vi "uploadBLE.vi"(11 "Queue in":refnum<queue>) -> ()   [LabVIEW 2022 SP3]
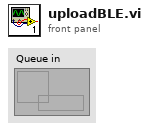
[diagram p1: front panel]
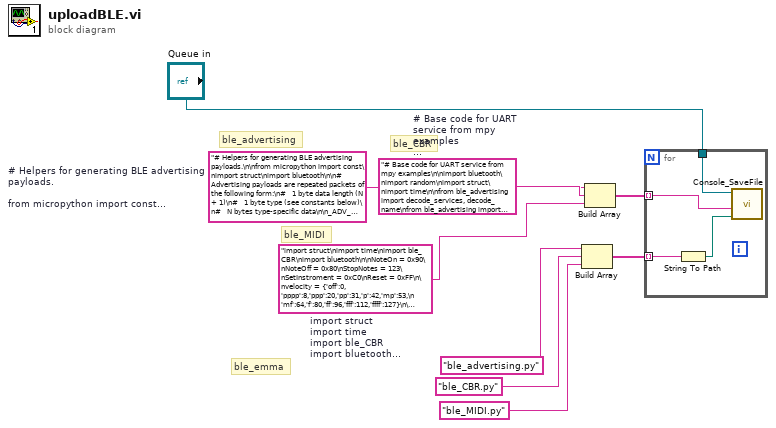
[diagram p0: block diagram]
diagram:
  w8 = "import struct\nimport time\nimport ble_CBR\nimport bluetooth\n\nNoteOn = 0x90\nNoteOff = 0x80\nStopNotes = 123\nSetInstroment = 0xC0\nReset = 0xFF\n\nvelocity = {'off':0, 'pppp':8,'ppp':20,'pp':31,'p':42,'mp':53,\n    'mf':64,'f':80,'ff':96,'fff':112,'ffff':127}\n\ninstruments = {'Acoustic Grand Piano':0,'Bright Acoustic Piano':1,'Electric Grand Piano':2,'Honky-tonk Piano':3,'Rhodes Piano':4,'Chorused Piano':5,'Harpsichord':6,'Clavinet':7,'Celesta':8,'Glockenspiel':9,'Music box':10,'Vibraphone':11,'Marimba':12,'Xylophone':13,'Tubular Bells':14,'Dulcimer':15,'Hammond Organ':16,'Percussive Organ':17,'Rock Organ':18,'Church Organ':19,\n    'Reed Organ':20,'Accordion':21,'Harmonica':22,'Tango Accordion':23,'Acoustic Guitar (nylon)':24,'Acoustic Guitar (steel)':25,'Electric Guitar (jazz)':26,'Electric Guitar (clean)':27,'Electric Guitar (muted)':28,'Overdriven Guitar':29,'Distortion Guitar':30,'Guitar Harmonics':31,'Acoustic Bass':32,'Electric Bass (finger)':33,'Electric Bass (pick)':34,'Fretless Bass':35,\n    'Slap Bass 1':36,'Slap Bass 2':37,'Synth Bass 1':38,'Synth Bass 2':39,'Violin':40,'Viola':41,'Cello':42,'Contrabass':43,'Tremolo Strings':44,'Pizzicato Strings':45,'Orchestral Harp':46,'Timpani':47,'String Ensemble 1':48,'String Ensemble 2':49,'Synth Strings 1':50,'Synth Strings 2':51,'Choir Aahs':52,'Voice Oohs':53,'Synth Voice':54,'Orchestra Hit':55,'Trumpet':56,\n    'Trombone':57,'Tuba':58,'Muted Trumpet':59,'French Horn':60,'Brass Section':61,'Synth Brass 1':62,'Synth Brass 2':63,'Soprano Sax':64,'Alto Sax':65,'Tenor Sax':66,'Baritone Sax':67,'Oboe':68,'English Horn':69,'Bassoon':70,'Clarinet':71,'Piccolo':72,'Flute':73,'Recorder':74,'Pan Flute':75,'Bottle Blow':76,'Shakuhachi':77,'Whistle':78,'Ocarina':79,'Lead 1 (square)':80,\n    'Lead 2 (sawtooth)':81,'Lead 3 (calliope lead)':82,'Lead 4 (chiffer lead)':83,'Lead 5 (charang)':84,'Lead 6 (voice)':85,'Lead 7 (fifths)':86,'Lead 8 (brass + lead)':87,'Pad 1 (new age)':88,'Pad 2 (warm)':89,'Pad 3 (polysynth)':90,'Pad 4 (choir)':91,'Pad 5 (bowed)':92,'Pad 6 (metallic)':93,'Pad 7 (halo)':94,'Pad 8 (sweep)':95,'FX 1 (rain)':96,'FX 2 (soundtrack)':97,\n    'FX 3 (crystal)':98,'FX 4 (atmosphere)':99,'FX 5 (brightness)':100,'FX 6 (goblins)':101,'FX 7 (echoes)':102,'FX 8 (sci-fi)':103,'Sitar':104,'Banjo':105,'Shamisen':106,'Koto':107,'Kalimba':108,'Bagpipe':109,'Fiddle':110,'Shana':111,'Tinkle Bell':112,'Agogo':113,'Steel Drums':114,'Woodblock':115,'Taiko Drum':116,'Melodic Tom':117,'Synth Drum':118,'Reverse Cymbal':119,\n    'Guitar Fret Noise':120,'Breath Noise':121,'Seashore':122,'Bird Tweet':123,'Telephone Ring':124,'Helicopter':125,'Applause':126,'Gunshot':127}\n\nclass MIDI_Player:\n    def __init__(self, name = 'MySpike'):\n        ble = bluetooth.BLE()\n        self.name = name\n        self.p = ble_CBR.BLESimplePeripheral(ble, 'MIDI', self.name)\n        self.p.on_write(self.on_rx)\n        \n    def on_rx(self,v):\n        print(\"RX\", v)\n        \n    def reset(self):\n        payload = struct.pack('b',Reset)\n        self.p.send(payload)   \n        \n    def wait_for_connection(self):\n        print('Waiting ',end = '')\n        while not self.is_connected():\n            print('.',end = '')\n            time.sleep(0.5)\n        self.reset()\n        print('success')     \n        \n    def is_connected(self):\n        return self.p.is_connected()\n        \n    def send(self, value):\n        if self.is_connected():\n            self.p.send(value)\n            return True\n        return False\n        \n    def fit(self, x):\n        return (0 if x < 0 else 127 if x > 127 else x)\n        \n    def sendPackage(self, cmd, notes, channel, verbose = False):\n        channel = 0x0F & channel\n        timestamp_ms = time.ticks_ms()\n        tsM = (timestamp_ms >> 7 & 0b111111) | 0x80\n        tsL =  0x80 | (timestamp_ms & 0b1111111)\n        c =  cmd | channel\n        payload = struct.pack('bb',tsM,tsL)\n        for note in notes:\n            payload += struct.pack('b',c)\n            for n in list(note):  # note should be a tuple\n                payload += struct.pack('b',self.fit(n))  # some commands are 1 byte, others 2\n        if verbose:\n            print([hex(i) for i in payload])\n        return self.send(payload)\n\n    def instrument(self, value = 57, channel = 0):\n        self.sendPackage(SetInstroment, [(value,),], channel)\n        \n    def disconnect(self):\n        self.p.disconnect()\n        \nclass MIDI_Instrument:\n    def __init__(self, midi, number=0, channel=0, verbose = False):\n        self.midi = midi\n        self.number = number\n        self.channel = channel\n        self.noteHistory = []\n        self.volume = 0\n        self.verbose = verbose\n        self.midi.instrument(number,channel)\n        \n    def on(self, note, vel = velocity['f']):\n        if type(note) == list:\n            self.chord(note,vel)\n        else:\n            self.midi.sendPackage(NoteOn, [(note, vel),], self.channel, self.verbose)\n            self.noteHistory.append(note)\n        \n    def chord(self, notes, vels = None):\n        if vels:\n            if type(vels) == list:\n                c = list(zip(notes,vels))\n            else:\n                c = [(note,vels) for note in notes]\n        else:\n            c = [(note,velocity['f']) for note in notes]\n        if self.verbose:\n            print(c)\n        self.midi.sendPackage(NoteOn, c, self.channel, self.verbose)\n        self.noteHistory.extend(notes)\n\n    def _off(self, note, vel):\n        self.midi.sendPackage(NoteOff, [(note, vel),], self.channel, self.verbose)\n        if note in self.noteHistory:\n            self.noteHistory.reverse()\n            self.noteHistory.pop(self.noteHistory.index(note))\n            self.noteHistory.reverse()  \n            if self.verbose:\n                print('deleted %d'%note)\n    \n    def off(self, note = None , vel = velocity['off']):\n        if note:\n            if type(note) == list:\n                for n in note:\n                    self._off(n, vel)\n            else:\n                self._off(note, vel)\n        else:\n            temp = self.noteHistory * 1 # force memory reallocation\n            for n in temp:\n                self._off(n, vel)\n            \n    def Stop(self):\n        self.midi.sendPackage(StopNotes, [], self.channel, self.verbose)\n      "  # import struct import time import ble_CBR import bluetooth  NoteOn = 0x90 NoteOff = 0x80 StopNotes = 123 SetInstroment = 0xC0 Reset = 0xFF  velocity = {'off':0, 'pppp':8,'ppp':20,'pp':31,'p':42,'mp':53,     'mf':64,'f':80,'ff':96,'fff':112,'ffff':127}  instruments = {'Acoustic Grand Piano':0,'Bright Acoustic Piano':1,'Electric Grand Piano':2,'Honky-tonk Piano':3,'Rhodes Piano':4,'Chorused Piano':5,'Harpsichord':6,'Clavinet':7,'Celesta':8,'Glockenspiel':9,'Music box':10,'Vibraphone':11,'Marimba':12,'Xylophone':13,'Tubular Bells':14,'Dulcimer':15,'Hammond Organ':16,'Percussive Organ':17,'Rock Organ':18,'Church Organ':19,     'Reed Organ':20,'Accordion':21,'Harmonica':22,'Tango Accordion':23,'Acoustic Guitar (nylon)':24,'Acoustic Guitar (steel)':25,'Electric Guitar (jazz)':26,'Electric Guitar (clean)':27,'Electric Guitar (muted)':28,'Overdriven Guitar':29,'Distortion Guitar':30,'Guitar Harmonics':31,'Acoustic Bass':32,'Electric Bass (finger)':33,'Electric Bass (pick)':34,'Fretless Bass':35,     'Slap Bass 1':36,'Slap Bass 2':37,'Synth Bass 1':38,'Synth Bass 2':39,'Violin':40,'Viola':41,'Cello':42,'Contrabass':43,'Tremolo Strings':44,'Pizzicato Strings':45,'Orchestral Harp':46,'Timpani':47,'String Ensemble 1':48,'String Ensemble 2':49,'Synth Strings 1':50,'Synth Strings 2':51,'Choir Aahs':52,'Voice Oohs':53,'Synth Voice':54,'Orchestra Hit':55,'Trumpet':56,     'Trombone':57,'Tuba':58,'Muted Trumpet':59,'French Horn':60,'Brass Section':61,'Synth Brass 1':62,'Synth Brass 2':63,'Soprano Sax':64,'Alto Sax':65,'Tenor Sax':66,'Baritone Sax':67,'Oboe':68,'English Horn':69,'Bassoon':70,'Clarinet':71,'Piccolo':72,'Flute':73,'Recorder':74,'Pan Flute':75,'Bottle Blow':76,'Shakuhachi':77,'Whistle':78,'Ocarina':79,'Lead 1 (square)':80,     'Lead 2 (sawtooth)':81,'Lead 3 (calliope lead)':82,'Lead 4 (chiffer lead)':83,'Lead 5 (charang)':84,'Lead 6 (voice)':85,'Lead 7 (fifths)':86,'Lead 8 (brass + lead)':87,'Pad 1 (new age)':88,'Pad 2 (warm)':89,'Pad 3 (polysynth)':90,'Pad 4 (choir)':91,'Pad 5 (bowed)':92,'Pad 6 (metallic)':93,'Pad 7 (halo)':94,'Pad 8 (sweep)':95,'FX 1 (rain)':96,'FX 2 (soundtrack)':97,     'FX 3 (crystal)':98,'FX 4 (atmosphere)':99,'FX 5 (brightness)':100,'FX 6 (goblins)':101,'FX 7 (echoes)':102,'FX 8 (sci-fi)':103,'Sitar':104,'Banjo':105,'Shamisen':106,'Koto':107,'Kalimba':108,'Bagpipe':109,'Fiddle':110,'Shana':111,'Tinkle Bell':112,'Agogo':113,'Steel Drums':114,'Woodblock':115,'Taiko Drum':116,'Melodic Tom':117,'Synth Drum':118,'Reverse Cymbal':119,     'Guitar Fret Noise':120,'Breath Noise':121,'Seashore':122,'Bird Tweet':123,'Telephone Ring':124,'Helicopter':125,'Applause':126,'Gunshot':127}  class MIDI_Player:     def __init__(self, name = 'MySpike'):         ble = bluetooth.BLE()         self.name = name         self.p = ble_CBR.BLESimplePeripheral(ble, 'MIDI', self.name)         self.p.on_write(self.on_rx)              def on_rx(self,v):         print("RX", v)              def reset(self):         payload = struct.pack('b',Reset)         self.p.send(payload)                 def wait_for_connection(self):         print('Waiting ',end = '')         while not self.is_connected():             print('.',end = '')             time.sleep(0.5)         self.reset()         print('success')                   def is_connected(self):         return self.p.is_connected()              def send(self, value):         if self.is_connected():             self.p.send(value)             return True         return False              def fit(self, x):         return (0 if x < 0 else 127 if x > 127 else x)              def sendPackage(self, cmd, notes, channel, verbose = False):         channel = 0x0F & channel         timestamp_ms = time.ticks_ms()         tsM = (timestamp_ms >> 7 & 0b111111) | 0x80         tsL =  0x80 | (timestamp_ms & 0b1111111)         c =  cmd | channel         payload = struct.pack('bb',tsM,tsL)         for note in notes:             payload += struct.pack('b',c)             for n in list(note):  # note should be a tuple                 payload += struct.pack('b',self.fit(n))  # some commands are 1 byte, others 2         if verbose:             print([hex(i) for i in payload])         return self.send(payload)      def instrument(self, value = 57, channel = 0):         self.sendPackage(SetInstroment, [(value,),], channel)              def disconnect(self):         self.p.disconnect()          class MIDI_Instrument:     def __init__(self, midi, number=0, channel=0, verbose = False):         self.midi = midi         self.number = number         self.channel = channel         self.noteHistory = []         self.volume = 0         self.verbose = verbose         self.midi.instrument(number,channel)              def on(self, note, vel = velocity['f']):         if type(note) == list:             self.chord(note,vel)         else:             self.midi.sendPackage(NoteOn, [(note, vel),], self.channel, self.verbose)             self.noteHistory.append(note)              def chord(self, notes, vels = None):         if vels:             if type(vels) == list:                 c = list(zip(notes,vels))             else:                 c = [(note,vels) for note in notes]         else:             c = [(note,velocity['f']) for note in notes]         if self.verbose:             print(c)         self.midi.sendPackage(NoteOn, c, self.channel, self.verbose)         self.noteHistory.extend(notes)      def _off(self, note, vel):         self.midi.sendPackage(NoteOff, [(note, vel),], self.channel, self.verbose)         if note in self.noteHistory:             self.noteHistory.reverse()             self.noteHistory.pop(self.noteHistory.index(note))             self.noteHistory.reverse()               if self.verbose:                 print('deleted %d'%note)          def off(self, note = None , vel = velocity['off']):         if note:             if type(note) == list:                 for n in note:                     self._off(n, vel)             else:                 self._off(note, vel)         else:             temp = self.noteHistory * 1 # force memory reallocation             for n in temp:                 self._off(n, vel)                  def Stop(self):         self.midi.sendPackage(StopNotes, [], self.channel, self.verbose)
  w7 = "# Base code for UART service from mpy examples\n\nimport bluetooth\nimport random\nimport struct\nimport time\n\nfrom ble_advertising import decode_services, decode_name\nfrom ble_advertising import advertising_payload\n\n_IRQ_CENTRAL_CONNECT = 1\n_IRQ_CENTRAL_DISCONNECT = 2\n_IRQ_GATTS_WRITE = 3\n_IRQ_GATTS_READ_REQUEST = 4\n_IRQ_SCAN_RESULT = 5\n_IRQ_SCAN_DONE = 6\n_IRQ_PERIPHERAL_CONNECT = 7\n_IRQ_PERIPHERAL_DISCONNECT = 8\n_IRQ_GATTC_SERVICE_RESULT = 9\n_IRQ_GATTC_SERVICE_DONE = 10\n_IRQ_GATTC_CHARACTERISTIC_RESULT = 11\n_IRQ_GATTC_CHARACTERISTIC_DONE = 12\n_IRQ_GATTC_DESCRIPTOR_RESULT = 13\n_IRQ_GATTC_DESCRIPTOR_DONE = 14\n_IRQ_GATTC_READ_RESULT = 15\n_IRQ_GATTC_READ_DONE = 16\n_IRQ_GATTC_WRITE_DONE = 17\n_IRQ_GATTC_NOTIFY = 18\n_IRQ_GATTC_INDICATE = 19\n\n_ADV_IND = 0x00\n_ADV_DIRECT_IND = 0x01\n_ADV_SCAN_IND = 0x02\n_ADV_NONCONN_IND = 0x03\n\n_UART_SERVICE_UUID = bluetooth.UUID(\"6E400001-B5A3-F393-E0A9-E50E24DCCA9E\")\n_UART_RX_CHAR_UUID = bluetooth.UUID(\"6E400002-B5A3-F393-E0A9-E50E24DCCA9E\")\n_UART_TX_CHAR_UUID = bluetooth.UUID(\"6E400003-B5A3-F393-E0A9-E50E24DCCA9E\")\n\n_FLAG_READ = 0x0002\n_FLAG_WRITE_NO_RESPONSE = 0x0004\n_FLAG_WRITE = 0x0008\n_FLAG_NOTIFY = 0x0010\n\n_UART_UUID = _UART_SERVICE_UUID\n_UART_TX = (_UART_TX_CHAR_UUID, _FLAG_READ | _FLAG_NOTIFY,)\n_UART_RX = (_UART_RX_CHAR_UUID, _FLAG_WRITE | _FLAG_WRITE_NO_RESPONSE,)\n_UART_SERVICE = (_UART_UUID,(_UART_TX, _UART_RX),)\n\n_MIDI_SERVICE_UUID = bluetooth.UUID(\"03B80E5A-EDE8-4B33-A751-6CE34EC4C700\")\n_MIDI_CHAR_UUID = bluetooth.UUID(\"7772E5DB-3868-4112-A1A9-F2669D106BF3\")\n\n_MIDI_UUID = _MIDI_SERVICE_UUID\n_MIDI_TXRX = (_MIDI_CHAR_UUID, _FLAG_READ | _FLAG_NOTIFY | _FLAG_WRITE_NO_RESPONSE,)\n_MIDI_SERVICE = (_MIDI_UUID,(_MIDI_TXRX,),)\n\n#------------------------------------Peripheral-------------------------------\n\nclass BLESimplePeripheral:\n    def __init__(self, ble, type = 'UART', name=\"SPIKE\"):\n        self.type = type\n        services = [_UART_UUID] if type == 'UART' else [_MIDI_UUID]\n        self._ble = ble\n        self._ble.active(True)\n        self._ble.irq(self._irq)\n        if self.type == 'UART':\n            ((self._handle_tx, self._handle_rx),) = self._ble.gatts_register_services((_UART_SERVICE,))\n            services = [_UART_UUID]\n            print('setup as uart')\n        else:\n            ((self._handle_tx, ),) = self._ble.gatts_register_services((_MIDI_SERVICE,))\n            self._handle_rx = self._handle_tx   # same handle for both directions\n            services = [_MIDI_UUID]\n            print('setup as midi')\n        self._connections = set()\n        self._write_callback = None\n        self._payload = advertising_payload(name=name, services=services)\n        self._advertise()\n\n    def _irq(self, event, data):\n        # Track connections so we can send notifications.\n        if event == _IRQ_CENTRAL_CONNECT:\n            conn_handle, _, _ = data\n            print(\"New connection\", conn_handle)\n            self._connections.add(conn_handle)\n        elif event == _IRQ_CENTRAL_DISCONNECT:\n            conn_handle, _, _ = data\n            print(\"Disconnected\", conn_handle)\n            self._connections.remove(conn_handle)\n            self._write_callback = None\n            # Start advertising again to allow a new connection.\n            #self._advertise()\n        elif event == _IRQ_GATTS_WRITE:\n            conn_handle, value_handle = data\n            value = self._ble.gatts_read(value_handle)\n            if value_handle == self._handle_rx and self._write_callback:\n                self._write_callback(value)\n\n    def send(self, data):\n        for conn_handle in self._connections:\n            self._ble.gatts_notify(conn_handle, self._handle_tx, data)\n\n    def is_connected(self):\n        return len(self._connections) > 0\n\n    def _advertise(self, interval_us=500000):\n        print(\"Starting advertising\")\n        self._ble.gap_advertise(interval_us, adv_data=self._payload)\n\n    def on_write(self, callback):\n        self._write_callback = callback\n        \n    def disconnect(self):\n        for conn_handle in self._connections:\n            self._ble.gap_disconnect(conn_handle)\n\n#------------------------------------Central-------------------------------\n\nclass BLESimpleCentral:     #only for UART - all midi is peripheral\n    def __init__(self, ble): \n        self._ble = ble\n        self._ble.active(True)\n        self._ble.irq(self._irq)\n\n        self._reset()\n\n    def _reset(self):\n        # Cached name and address from a successful scan.\n        self._name = None\n        self._addr_type = None\n        self._addr = None\n\n        # Callbacks for completion of various operations.\n        # These reset back to None after being invoked.\n        self._scan_callback = None\n        self._conn_callback = None\n        self._read_callback = None\n\n        # Persistent callback for when new data is notified from the device.\n        self._notify_callback = None\n\n        # Connected device.\n        self._conn_handle = None\n        self._start_handle = None\n        self._end_handle = None\n        self._tx_handle = None\n        self._rx_handle = None\n\n    def _irq(self, event, data):\n        if event == _IRQ_SCAN_RESULT:\n            addr_type, addr, adv_type, rssi, adv_data = data\n            if adv_type in (_ADV_IND, _ADV_DIRECT_IND) and _UART_SERVICE_UUID in decode_services(adv_data):\n                # Found a potential device, remember it and stop scanning.\n                self._addr_type = addr_type\n                self._addr = bytes(addr)  # Note: addr buffer is owned by caller so need to copy it.\n                self._name = decode_name(adv_data) or \"?\"\n                self._ble.gap_scan(None)\n\n        elif event == _IRQ_SCAN_DONE:\n            if self._scan_callback:\n                if self._addr:\n                    # Found a device during the scan (and the scan was explicitly stopped).\n                    self._scan_callback(self._addr_type, self._addr, self._name)\n                    self._scan_callback = None\n                else:\n                    # Scan timed out.\n                    self._scan_callback(None, None, None)\n\n        elif event == _IRQ_PERIPHERAL_CONNECT:\n            # Connect successful.\n            conn_handle, addr_type, addr = data\n            if addr_type == self._addr_type and addr == self._addr:\n                self._conn_handle = conn_handle\n                self._ble.gattc_discover_services(self._conn_handle)\n\n        elif event == _IRQ_PERIPHERAL_DISCONNECT:\n            # Disconnect (either initiated by us or the remote end).\n            conn_handle, _, _ = data\n            if conn_handle == self._conn_handle:\n                # If it was initiated by us, it'll already be reset.\n                self._reset()\n\n        elif event == _IRQ_GATTC_SERVICE_RESULT:\n            # Connected device returned a service.\n            conn_handle, start_handle, end_handle, uuid = data\n            print(\"service\", data)\n            if conn_handle == self._conn_handle and uuid == _UART_SERVICE_UUID:\n                self._start_handle, self._end_handle = start_handle, end_handle\n\n        elif event == _IRQ_GATTC_SERVICE_DONE:\n            # Service query complete.\n            if self._start_handle and self._end_handle:\n                self._ble.gattc_discover_characteristics(self._conn_handle, self._start_handle, self._end_handle)\n            else:\n                print(\"Failed to find uart service.\")\n\n        elif event == _IRQ_GATTC_CHARACTERISTIC_RESULT:\n            # Connected device returned a characteristic.\n            conn_handle, def_handle, value_handle, properties, uuid = data\n            if conn_handle == self._conn_handle and uuid == _UART_RX_CHAR_UUID:\n                self._rx_handle = value_handle\n            if conn_handle == self._conn_handle and uuid == _UART_TX_CHAR_UUID:\n                self._tx_handle = value_handle\n\n        elif event == _IRQ_GATTC_CHARACTERISTIC_DONE:\n            # Characteristic query complete.\n            if self._tx_handle is not None and self._rx_handle is not None:\n                # We've finished connecting and discovering device, fire the connect callback.\n                if self._conn_callback:\n                    self._conn_callback()\n            else:\n                print(\"Failed to find uart rx characteristic.\")\n\n        elif event == _IRQ_GATTC_WRITE_DONE:\n            conn_handle, value_handle, status = data\n            print(\"TX complete\")\n\n        elif event == _IRQ_GATTC_NOTIFY:\n            conn_handle, value_handle, notify_data = data\n            if conn_handle == self._conn_handle and value_handle == self._tx_handle:\n                if self._notify_callback:\n                    self._notify_callback(notify_data)\n\n    # Returns true if we've successfully connected and discovered characteristics.\n    def is_connected(self):\n        return (self._conn_handle is not None and self._tx_handle is not None and self._rx_handle is not None)\n\n    # Find a device advertising the environmental sensor service.\n    def scan(self, callback=None):\n        self._addr_type = None\n        self._addr = None\n        self._scan_callback = callback\n        self._ble.gap_scan(2000, 30000, 30000)\n\n    # Connect to the specified device (otherwise use cached address from a scan).\n    def connect(self, addr_type=None, addr=None, callback=None):\n        self._addr_type = addr_type or self._addr_type\n        self._addr = addr or self._addr\n        self._conn_callback = callback\n        if self._addr_type is None or self._addr is None:\n            return False\n        self._ble.gap_connect(self._addr_type, self._addr)\n        return True\n\n    # Disconnect from current device.\n    def disconnect(self):\n        if not self._conn_handle:\n            return\n        self._ble.gap_disconnect(self._conn_handle)\n        self._reset()\n\n    # Send data over the UART\n    def write(self, v, response=False):\n        if not self.is_connected():\n            return\n        self._ble.gattc_write(self._conn_handle, self._rx_handle, v, 1 if response else 0)\n\n    # Set handler for when data is received over the UART.\n    def on_notify(self, callback):\n        self._notify_callback = callback"  # # Base code for UART service from mpy examples  import bluetooth import random import struct import time  from ble_advertising import decode_services, decode_name from ble_advertising import advertising_payload  _IRQ_CENTRAL_CONNECT = 1 _IRQ_CENTRAL_DISCONNECT = 2 _IRQ_GATTS_WRITE = 3 _IRQ_GATTS_READ_REQUEST = 4 _IRQ_SCAN_RESULT = 5 _IRQ_SCAN_DONE = 6 _IRQ_PERIPHERAL_CONNECT = 7 _IRQ_PERIPHERAL_DISCONNECT = 8 _IRQ_GATTC_SERVICE_RESULT = 9 _IRQ_GATTC_SERVICE_DONE = 10 _IRQ_GATTC_CHARACTERISTIC_RESULT = 11 _IRQ_GATTC_CHARACTERISTIC_DONE = 12 _IRQ_GATTC_DESCRIPTOR_RESULT = 13 _IRQ_GATTC_DESCRIPTOR_DONE = 14 _IRQ_GATTC_READ_RESULT = 15 _IRQ_GATTC_READ_DONE = 16 _IRQ_GATTC_WRITE_DONE = 17 _IRQ_GATTC_NOTIFY = 18 _IRQ_GATTC_INDICATE = 19  _ADV_IND = 0x00 _ADV_DIRECT_IND = 0x01 _ADV_SCAN_IND = 0x02 _ADV_NONCONN_IND = 0x03  _UART_SERVICE_UUID = bluetooth.UUID("6E400001-B5A3-F393-E0A9-E50E24DCCA9E") _UART_RX_CHAR_UUID = bluetooth.UUID("6E400002-B5A3-F393-E0A9-E50E24DCCA9E") _UART_TX_CHAR_UUID = bluetooth.UUID("6E400003-B5A3-F393-E0A9-E50E24DCCA9E")  _FLAG_READ = 0x0002 _FLAG_WRITE_NO_RESPONSE = 0x0004 _FLAG_WRITE = 0x0008 _FLAG_NOTIFY = 0x0010  _UART_UUID = _UART_SERVICE_UUID _UART_TX = (_UART_TX_CHAR_UUID, _FLAG_READ | _FLAG_NOTIFY,) _UART_RX = (_UART_RX_CHAR_UUID, _FLAG_WRITE | _FLAG_WRITE_NO_RESPONSE,) _UART_SERVICE = (_UART_UUID,(_UART_TX, _UART_RX),)  _MIDI_SERVICE_UUID = bluetooth.UUID("03B80E5A-EDE8-4B33-A751-6CE34EC4C700") _MIDI_CHAR_UUID = bluetooth.UUID("7772E5DB-3868-4112-A1A9-F2669D106BF3")  _MIDI_UUID = _MIDI_SERVICE_UUID _MIDI_TXRX = (_MIDI_CHAR_UUID, _FLAG_READ | _FLAG_NOTIFY | _FLAG_WRITE_NO_RESPONSE,) _MIDI_SERVICE = (_MIDI_UUID,(_MIDI_TXRX,),)  #------------------------------------Peripheral-------------------------------  class BLESimplePeripheral:     def __init__(self, ble, type = 'UART', name="SPIKE"):         self.type = type         services = [_UART_UUID] if type == 'UART' else [_MIDI_UUID]         self._ble = ble         self._ble.active(True)         self._ble.irq(self._irq)         if self.type == 'UART':             ((self._handle_tx, self._handle_rx),) = self._ble.gatts_register_services((_UART_SERVICE,))             services = [_UART_UUID]             print('setup as uart')         else:             ((self._handle_tx, ),) = self._ble.gatts_register_services((_MIDI_SERVICE,))             self._handle_rx = self._handle_tx   # same handle for both directions             services = [_MIDI_UUID]             print('setup as midi')         self._connections = set()         self._write_callback = None         self._payload = advertising_payload(name=name, services=services)         self._advertise()      def _irq(self, event, data):         # Track connections so we can send notifications.         if event == _IRQ_CENTRAL_CONNECT:             conn_handle, _, _ = data             print("New connection", conn_handle)             self._connections.add(conn_handle)         elif event == _IRQ_CENTRAL_DISCONNECT:             conn_handle, _, _ = data             print("Disconnected", conn_handle)             self._connections.remove(conn_handle)             self._write_callback = None             # Start advertising again to allow a new connection.             #self._advertise()         elif event == _IRQ_GATTS_WRITE:             conn_handle, value_handle = data             value = self._ble.gatts_read(value_handle)             if value_handle == self._handle_rx and self._write_callback:                 self._write_callback(value)      def send(self, data):         for conn_handle in self._connections:             self._ble.gatts_notify(conn_handle, self._handle_tx, data)      def is_connected(self):         return len(self._connections) > 0      def _advertise(self, interval_us=500000):         print("Starting advertising")         self._ble.gap_advertise(interval_us, adv_data=self._payload)      def on_write(self, callback):         self._write_callback = callback              def disconnect(self):         for conn_handle in self._connections:             self._ble.gap_disconnect(conn_handle)  #------------------------------------Central-------------------------------  class BLESimpleCentral:     #only for UART - all midi is peripheral     def __init__(self, ble):          self._ble = ble         self._ble.active(True)         self._ble.irq(self._irq)          self._reset()      def _reset(self):         # Cached name and address from a successful scan.         self._name = None         self._addr_type = None         self._addr = None          # Callbacks for completion of various operations.         # These reset back to None after being invoked.         self._scan_callback = None         self._conn_callback = None         self._read_callback = None          # Persistent callback for when new data is notified from the device.         self._notify_callback = None          # Connected device.         self._conn_handle = None         self._start_handle = None         self._end_handle = None         self._tx_handle = None         self._rx_handle = None      def _irq(self, event, data):         if event == _IRQ_SCAN_RESULT:             addr_type, addr, adv_type, rssi, adv_data = data             if adv_type in (_ADV_IND, _ADV_DIRECT_IND) and _UART_SERVICE_UUID in decode_services(adv_data):                 # Found a potential device, remember it and stop scanning.                 self._addr_type = addr_type                 self._addr = bytes(addr)  # Note: addr buffer is owned by caller so need to copy it.                 self._name = decode_name(adv_data) or "?"                 self._ble.gap_scan(None)          elif event == _IRQ_SCAN_DONE:             if self._scan_callback:                 if self._addr:                     # Found a device during the scan (and the scan was explicitly stopped).                     self._scan_callback(self._addr_type, self._addr, self._name)                     self._scan_callback = None                 else:                     # Scan timed out.                     self._scan_callback(None, None, None)          elif event == _IRQ_PERIPHERAL_CONNECT:             # Connect successful.             conn_handle, addr_type, addr = data             if addr_type == self._addr_type and addr == self._addr:                 self._conn_handle = conn_handle                 self._ble.gattc_discover_services(self._conn_handle)          elif event == _IRQ_PERIPHERAL_DISCONNECT:             # Disconnect (either initiated by us or the remote end).             conn_handle, _, _ = data             if conn_handle == self._conn_handle:                 # If it was initiated by us, it'll already be reset.                 self._reset()          elif event == _IRQ_GATTC_SERVICE_RESULT:             # Connected device returned a service.             conn_handle, start_handle, end_handle, uuid = data             print("service", data)             if conn_handle == self._conn_handle and uuid == _UART_SERVICE_UUID:                 self._start_handle, self._end_handle = start_handle, end_handle          elif event == _IRQ_GATTC_SERVICE_DONE:             # Service query complete.             if self._start_handle and self._end_handle:                 self._ble.gattc_discover_characteristics(self._conn_handle, self._start_handle, self._end_handle)             else:                 print("Failed to find uart service.")          elif event == _IRQ_GATTC_CHARACTERISTIC_RESULT:             # Connected device returned a characteristic.             conn_handle, def_handle, value_handle, properties, uuid = data             if conn_handle == self._conn_handle and uuid == _UART_RX_CHAR_UUID:                 self._rx_handle = value_handle             if conn_handle == self._conn_handle and uuid == _UART_TX_CHAR_UUID:                 self._tx_handle = value_handle          elif event == _IRQ_GATTC_CHARACTERISTIC_DONE:             # Characteristic query complete.             if self._tx_handle is not None and self._rx_handle is not None:                 # We've finished connecting and discovering device, fire the connect callback.                 if self._conn_callback:                     self._conn_callback()             else:                 print("Failed to find uart rx characteristic.")          elif event == _IRQ_GATTC_WRITE_DONE:             conn_handle, value_handle, status = data             print("TX complete")          elif event == _IRQ_GATTC_NOTIFY:             conn_handle, value_handle, notify_data = data             if conn_handle == self._conn_handle and value_handle == self._tx_handle:                 if self._notify_callback:                     self._notify_callback(notify_data)      # Returns true if we've successfully connected and discovered characteristics.     def is_connected(self):         return (self._conn_handle is not None and self._tx_handle is not None and self._rx_handle is not None)      # Find a device advertising the environmental sensor service.     def scan(self, callback=None):         self._addr_type = None         self._addr = None         self._scan_callback = callback         self._ble.gap_scan(2000, 30000, 30000)      # Connect to the specified device (otherwise use cached address from a scan).     def connect(self, addr_type=None, addr=None, callback=None):         self._addr_type = addr_type or self._addr_type         self._addr = addr or self._addr         self._conn_callback = callback         if self._addr_type is None or self._addr is None:             return False         self._ble.gap_connect(self._addr_type, self._addr)         return True      # Disconnect from current device.     def disconnect(self):         if not self._conn_handle:             return         self._ble.gap_disconnect(self._conn_handle)         self._reset()      # Send data over the UART     def write(self, v, response=False):         if not self.is_connected():             return         self._ble.gattc_write(self._conn_handle, self._rx_handle, v, 1 if response else 0)      # Set handler for when data is received over the UART.     def on_notify(self, callback):         self._notify_callback = callback
  w6 = "# Helpers for generating BLE advertising payloads.\n\nfrom micropython import const\nimport struct\nimport bluetooth\n\n# Advertising payloads are repeated packets of the following form:\n#   1 byte data length (N + 1)\n#   1 byte type (see constants below)\n#   N bytes type-specific data\n\n_ADV_TYPE_FLAGS = const(0x01)\n_ADV_TYPE_NAME = const(0x09)\n_ADV_TYPE_UUID16_COMPLETE = const(0x3)\n_ADV_TYPE_UUID32_COMPLETE = const(0x5)\n_ADV_TYPE_UUID128_COMPLETE = const(0x7)\n_ADV_TYPE_UUID16_MORE = const(0x2)\n_ADV_TYPE_UUID32_MORE = const(0x4)\n_ADV_TYPE_UUID128_MORE = const(0x6)\n_ADV_TYPE_APPEARANCE = const(0x19)\n\n\n# Generate a payload to be passed to gap_advertise(adv_data=...).\ndef advertising_payload(limited_disc=False, br_edr=False, name=None, services=None, appearance=0):\n    payload = bytearray()\n\n    def _append(adv_type, value):\n        nonlocal payload\n        payload += struct.pack(\"BB\", len(value) + 1, adv_type) + value\n\n    _append(_ADV_TYPE_FLAGS,struct.pack(\"B\", (0x01 if limited_disc else 0x02) + (0x18 if br_edr else 0x04)),)\n\n    if name:\n        _append(_ADV_TYPE_NAME, name)\n\n    if services:\n        for uuid in services:\n            b = bytes(uuid)\n            if len(b) == 2:\n                _append(_ADV_TYPE_UUID16_COMPLETE, b)\n            elif len(b) == 4:\n                _append(_ADV_TYPE_UUID32_COMPLETE, b)\n            elif len(b) == 16:\n                _append(_ADV_TYPE_UUID128_COMPLETE, b)\n\n    # See org.bluetooth.characteristic.gap.appearance.xml\n    if appearance:\n        _append(_ADV_TYPE_APPEARANCE, struct.pack(\"<h\", appearance))\n\n    return payload\n\n\ndef decode_field(payload, adv_type):\n    i = 0\n    result = []\n    while i + 1 < len(payload):\n        if payload[i + 1] == adv_type:\n            result.append(payload[i + 2 : i + payload[i] + 1])\n        i += 1 + payload[i]\n    return result\n\n\ndef decode_name(payload):\n    n = decode_field(payload, _ADV_TYPE_NAME)\n    return str(n[0], \"utf-8\") if n else \"\"\n\n\ndef decode_services(payload):\n    services = []\n    for u in decode_field(payload, _ADV_TYPE_UUID16_COMPLETE):\n        services.append(bluetooth.UUID(struct.unpack(\"<h\", u)[0]))\n    for u in decode_field(payload, _ADV_TYPE_UUID32_COMPLETE):\n        services.append(bluetooth.UUID(struct.unpack(\"<d\", u)[0]))\n    for u in decode_field(payload, _ADV_TYPE_UUID128_COMPLETE):\n        services.append(bluetooth.UUID(u))\n    return services\n\n\ndef demo():\n    payload = advertising_payload(name=\"mp2\",services=[bluetooth.UUID(0x181A), bluetooth.UUID(\"6E400001-B5A3-F393-E0A9-E50E24DCCA9E\")],)\n    print(payload)\n    print(decode_name(payload))\n    print(decode_services(payload))\n\n\nif __name__ == \"__main__\":\n    demo()\n\n"  # # Helpers for generating BLE advertising payloads.  from micropython import const import struct import bluetooth  # Advertising payloads are repeated packets of the following form: #   1 byte data length (N + 1) #   1 byte type (see constants below) #   N bytes type-specific data  _ADV_TYPE_FLAGS = const(0x01) _ADV_TYPE_NAME = const(0x09) _ADV_TYPE_UUID16_COMPLETE = const(0x3) _ADV_TYPE_UUID32_COMPLETE = const(0x5) _ADV_TYPE_UUID128_COMPLETE = const(0x7) _ADV_TYPE_UUID16_MORE = const(0x2) _ADV_TYPE_UUID32_MORE = const(0x4) _ADV_TYPE_UUID128_MORE = const(0x6) _ADV_TYPE_APPEARANCE = const(0x19)   # Generate a payload to be passed to gap_advertise(adv_data=...). def advertising_payload(limited_disc=False, br_edr=False, name=None, services=None, appearance=0):     payload = bytearray()      def _append(adv_type, value):         nonlocal payload         payload += struct.pack("BB", len(value) + 1, adv_type) + value      _append(_ADV_TYPE_FLAGS,struct.pack("B", (0x01 if limited_disc else 0x02) + (0x18 if br_edr else 0x04)),)      if name:         _append(_ADV_TYPE_NAME, name)      if services:         for uuid in services:             b = bytes(uuid)             if len(b) == 2:                 _append(_ADV_TYPE_UUID16_COMPLETE, b)             elif len(b) == 4:                 _append(_ADV_TYPE_UUID32_COMPLETE, b)             elif len(b) == 16:                 _append(_ADV_TYPE_UUID128_COMPLETE, b)      # See org.bluetooth.characteristic.gap.appearance.xml     if appearance:         _append(_ADV_TYPE_APPEARANCE, struct.pack("<h", appearance))      return payload   def decode_field(payload, adv_type):     i = 0     result = []     while i + 1 < len(payload):         if payload[i + 1] == adv_type:             result.append(payload[i + 2 : i + payload[i] + 1])         i += 1 + payload[i]     return result   def decode_name(payload):     n = decode_field(payload, _ADV_TYPE_NAME)     return str(n[0], "utf-8") if n else ""   def decode_services(payload):     services = []     for u in decode_field(payload, _ADV_TYPE_UUID16_COMPLETE):         services.append(bluetooth.UUID(struct.unpack("<h", u)[0]))     for u in decode_field(payload, _ADV_TYPE_UUID32_COMPLETE):         services.append(bluetooth.UUID(struct.unpack("<d", u)[0]))     for u in decode_field(payload, _ADV_TYPE_UUID128_COMPLETE):         services.append(bluetooth.UUID(u))     return services   def demo():     payload = advertising_payload(name="mp2",services=[bluetooth.UUID(0x181A), bluetooth.UUID("6E400001-B5A3-F393-E0A9-E50E24DCCA9E")],)     print(payload)     print(decode_name(payload))     print(decode_services(payload))   if __name__ == "__main__":     demo()
  # "ble_emma"
  # "ble_MIDI"
  # "ble_CBR"
  # "ble_advertising"
  n1 = Build Array("ble_advertising.py", "ble_CBR.py", "ble_MIDI.py") -> (w2:string[])
  n2 = Build Array(w6, w7, w8) -> (w1:string[])
  n3 = for {
    tunnel: w1 -> [w13] mode=indexing
    tunnel: w2 -> [w12] mode=indexing
    tunnel: "Queue in" -> [w10]
    n4 = String To Path(string=w12) -> (path=w11:path)
    n5 = call "Console_SaveFile.vi"("Path"=w11, "Code"=w13, "Queue in"=w10) -> ()  [unwired: 9 in]
  }
